vi "Solutions AM Demodulation.vi"(9 "载波幅度":dbl, 10 "载波频率":dbl, 11 "AM 调制信号(时域)":waveform(dbl)) -> (3 "解调信号":waveform(dbl)(graph))   [LabVIEW 2015]
uses:
  <vilib>/measure/NI_MABase.lvlib
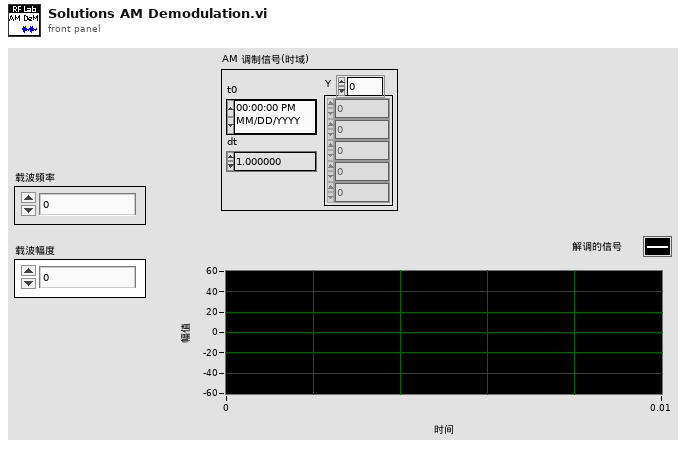
[diagram p1: front panel]
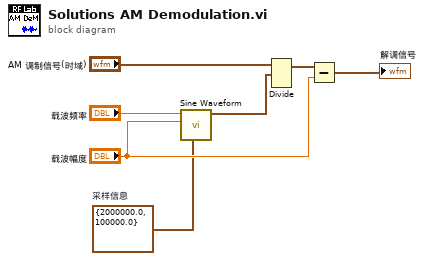
[diagram p0: block diagram]
diagram:
  w2 = cluster{"Fs":dbl, "#s":dbl} {"Fs"=2000000.0, "#s"=100000.0}  # 采样信息
  n1 = call <vilib>:"Sine Waveform.vi"("sampling info"=w2, "amplitude"="载波幅度", "frequency"="载波频率") -> ("signal out"=w5:waveform(dbl))  [unwired: 7 in, 1 out]
  n2 = Divide(1:w5, 2:"AM 调制信号(时域)") -> (0:w6:waveform(dbl))  [unwired: 1 in, 1 out]
  n3 = Subtract(x=w6, y="载波幅度") -> (x-y=→"解调信号":waveform(dbl))
